vi "PH_PowerUnit_BaseClass.destructor.vi"(0 "i ref in":refnum<vi>, 5 "error in(no error)":errorcluster) -> (19 "error out":errorcluster)   [LabVIEW 2014, in "PH_PowerUnit_BaseClass.lvlib"]
doc: "This is the destructor of a class.\n\nLicense Agreement for this software:\n\nCopyright (C)\nGesellschaft für Schwerionenforschung, GSI\nPlanckstr. 1\n64291 Darmstadt\nGermany\n\nContact: D.Beck@gsi.de \n\nThis program is free software; you can redistribute it and/or modify it under the terms of the \nGNU General Public License as published by the Free Software Foundation; either version 2 of \nthe license, or (at your option) any later version.\n\nThis program is distributed in the hope that it will be useful, but WITHOUT ANY WARRANTY; \nwithout even the implied warranty of MERCHANTABILITY or FITNESS FOR A PARTICULAR PURPOSE. See the GNU General License for more details (http://www.gnu.org).\n\nGesellschaft für Schwerionenforschung, GSI\nPlanckstr. 1, 64291 Darmstadt, Germany\nFor all questions and ideas contact: M.Richter@gsi.de, H.Brand@gsi.de or D.Beck@gsi.de.\nLast update: 16-JUN-2004"
uses:
  PH_PowerUnit_BaseClass.lvlib
  CSlibraries-extern/DimLVEvent/LVDimInterface/LVDimInterface.lvlib
  PH_PSDBWriter/PH_PSDBWriter.lvlib
  PH_SM_Class/PH_SM_Class.lvlib
  PH_StatusHandler/PH_StatusHandler.lvlib
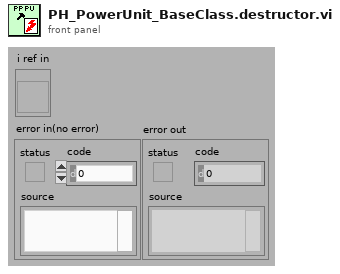
[diagram p1: front panel]
types:
  T1 = typedef "PH_PowerUnit_BaseClass.lvlib/PH_PowerUnit_BaseClass.i attribute.ctl" = cluster{"Constructor finished":bool, "PU":cluster{"In use":bool, "Service ID in use":i32, "GUI Ref":refnum<vi>}, "Enabling":cluster{"State":T2, "GUI Ref":refnum<vi>}, "Timing":cluster{"Last Shot":dbl, "Time between Shots [Sec]":dbl, "Waiting Time over?":bool, "Service ID Waiting Time":i32, "GUI Ref":refnum<vi>, "Instance":cluster{"Status":T3, "linked?":bool, "GUI Ref":refnum<vi>}}, "Sequencer":cluster{"SM State":string, "GUI Ref":refnum<vi>, "linked":bool}, "Subscribed Trendmssgs":cluster{"Tagname":string, "Status":T3, "linked?":bool, "Shot Condition":T3, "GUI Ref":refnum<vi>}[], "PP PU":T4, "Default Voltage (V)":dbl, "GUI Refs":T5, "PSDB data":cluster{"Shot Voltage [V]":dbl, "State TO SM":T6, "Write 2 early":bool}, "State TO SM":T6}
  T2 = typedef "PH_SystemInformation.lvlib/PH_SystemInformationEnabling State.ctl" = i32
  T3 = typedef "PH_StatusHandler.lvlib/PH_StatusHandler.Status.ctl" = i16
  T4 = typedef "PH_PP_Common.lvlib/PH_PP_Common.PUs.ctl" = enum16{"no Info", "PA-19mm-1", "PA-19mm-2", "PA-45mm-PILC", "PA-45mm-MAIN", "MA-PU-1", "MA-PU-2", "MA-PU-3", "MA-PU-4", "MA-PU-5", "MA-PU-6", "MA-FR", "MA-PILC", "PA-45mm-DP"}
  T5 = typedef "PH_PowerUnit_BaseClass.lvlib/PH_PowerUnit_BaseClass.GUI Refs.ctl" = cluster{"Delete Inst":refnum<vi>, "State TO SM":refnum<vi>, "State SM":refnum<vi>, "Fire":refnum<vi>}
  T6 = typedef "PH_PowerUnit_BaseClass.lvlib/PH_PowerUnit_BaseClass.SM States.ctl" = enum16{".", "Stand by", "Switch PU on", "Configure", "Set Default Voltage", "Set STANDBY", "Set READY", "Wait for Shot Cmd", "Open Dump Rods", "Open Ross Relais", "Close Ross Relais", "Switch PSU on", "Switch PSU off", "Charge", "Switch GD Channel on", "Close Dump Rods", "Rods-TO", "RR-TO", "PSU-TO", "Trigger-TO"}
  T7 = enum16{"SetAttribute", "GetAttribute", "CreateAttribute", "DestroyAttribute", "DestroyAllAtributes"}
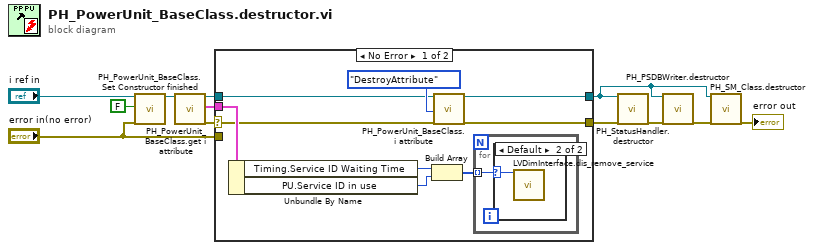
[diagram p0: block diagram]
diagram:
  n1 = call "PH_PowerUnit_BaseClass.Set Constructor finished.vi"("VI in"="i ref in", "Constructor finished"=FALSE, "error in (no error)"="error in(no error)") -> ("VI out"=w6:refnum<vi>)  [unwired: 15 in, 1 out]
  n2 = call "PH_PowerUnit_BaseClass.get i attribute.vi"("i ref in"=w6) -> ("i ref out"=w11:refnum<vi>, "i attribute"=w12:T1, "error out"=w10:errorcluster)  [unwired: 16 in]
  n3 = case shown="No Error" w10 {
    selector: w10 -> [w13 _]
    tunnel: w12 -> [w19 _]
    tunnel: w11 -> [w14 w25]
    tunnel: [w16 w25] -> w1
    tunnel: [w15 w24] -> w9
    tunnel: "error in(no error)" -> [_ w24]
    frame No Error {
      n4 = Unbundle By Name(w19) -> ("Timing.Service ID Waiting Time"=w20:i32, "PU.Service ID in use"=w17:i32)
      n5 = Build Array(w20, w17) -> (w21:i32[])
      n6 = call "PH_PowerUnit_BaseClass.i attribute.vi"("VI Refnum"=w14, "Action"=T7."DestroyAttribute", "error in (no error)"=w13) -> ("VI Refnum out"=w16:refnum<vi>, "error out"=w15:errorcluster)  [unwired: 14 in, 1 out]
      n7 = for {
        tunnel: w21 -> [w22] mode=indexing
        n8 = case shown="Default" w22 {
          selector: w22 -> [_ w23]
          frame -1 {
          }
          frame Default {
            n9 = call "LVDimInterface.dis_remove_service.vi"("my_serviceID"=w23) -> ()  [unwired: 18 in, 1 out]
          }
        }
      }
    }
    frame Error {
    }
  }
  n10 = call "PH_StatusHandler.destructor.vi"("i ref in"=w1, "error in(no error)"=w9) -> ("error out"=w2:errorcluster)  [unwired: 17 in]
  n11 = call "PH_PSDBWriter.destructor.vi"("i ref in"=w1, "error in(no error)"=w2) -> ("error out"=w4:errorcluster)  [unwired: 17 in]
  n12 = call "PH_SM_Class.destructor.vi"("i ref in"=w1, "error in(no error)"=w4) -> ("error out"=→"error out":errorcluster)  [unwired: 17 in]
